vi "ReadCom.vi"(10 "仪器名称":string, 11 "MyIndex":u8) -> (1 "Baudrate":i32, 2 "COM":string, 3 "OK?":bool)   [LabVIEW 2015]
uses:
  <vilib>/Utility/config.llb/Read Key (String).vi
  <vilib>/Utility/config.llb/NI_LVConfig.lvlib
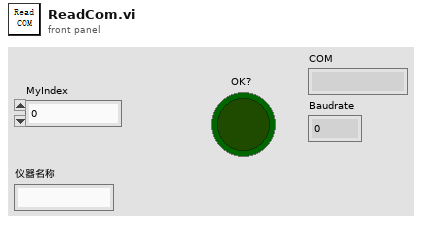
[diagram p1: front panel]
types:
  T1 = typedef "NI_LVConfig.lvlib/Config Data RefNum.ctl" = refnum<k1>
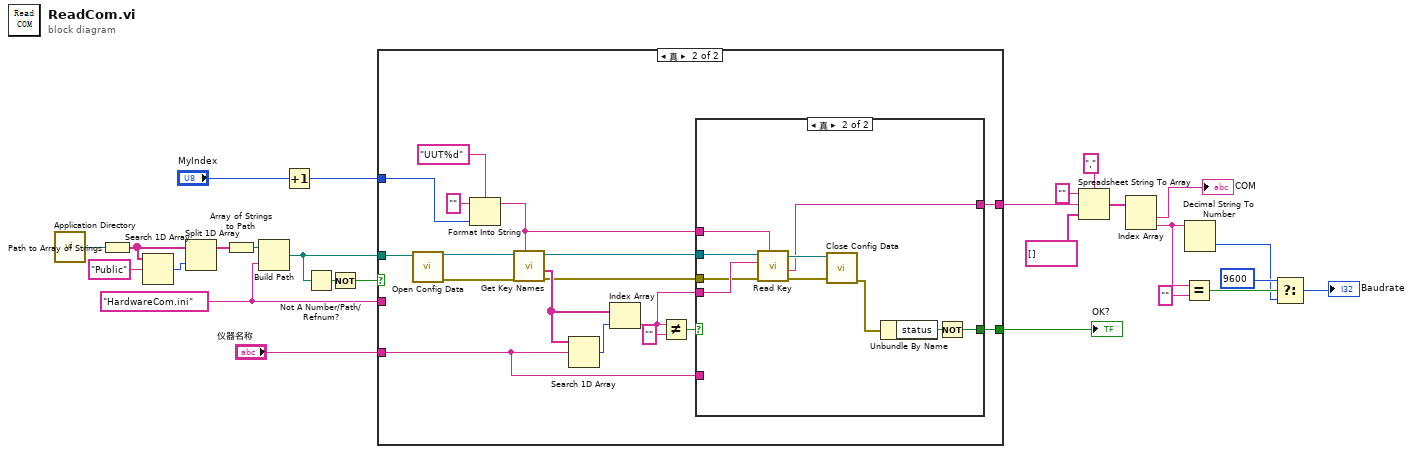
[diagram p0: block diagram]
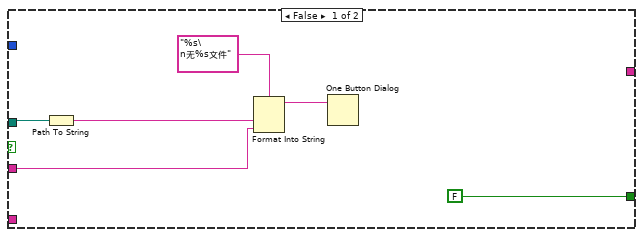
[diagram p2: hidden frame]
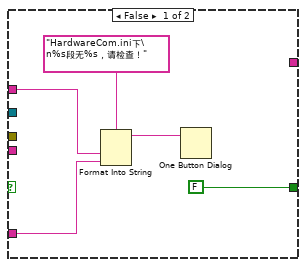
[diagram p3: hidden frame]
diagram:
  w14 = "HardwareCom.ini" ("名称或相对路径")
  n1 = call <vilib>:"Application Directory.vi"() -> ("Application Directory"=w26:path)
  n2 = Path to Array of Strings(0:w26) -> (2:w24:string[])  [unwired: 1 out]
  n3 = Search 1D Array(1D array=w24, element="Public" ("元素")) -> (index of element=w23:i32)  [unwired: 1 in]
  n4 = Split 1D Array(array=w24, index=w23) -> (first subarray=w22:string[])  [unwired: 1 out]
  n5 = Array of Strings to Path(0:w22) -> (2:w21:path)  [unwired: 1 in]
  n6 = Build Path(base path=w21, name or relative path=w14) -> (appended path=w18:path)
  n7 = Increment(x="MyIndex") -> (x+1=w15:u8)
  n8 = Not A Number/Path/Refnum?(number/path/refnum=w18) -> (NaN/Path/Refnum?=w20:bool)
  n9 = Not(x=w20) -> (.not. x?=w19:bool)
  n10 = case shown="真" w19 {
    tunnel: w18 -> [w31 w49]
    tunnel: w15 -> [_ w41]
    tunnel: "仪器名称" -> [_ w39]
    tunnel: w14 -> [w29 _]
    tunnel: [FALSE w37] -> w13
    tunnel: [_ w33] -> w11
    frame False {
      n11 = Path To String(path=w31) -> (string=w30:string)
      n12 = Format Into String(format string="%s\n无%s文件" ("消息"), w30, w29) -> (resulting string=w28:string)  [unwired: 2 in, 1 out]
      n13 = One Button Dialog(message=w28) -> ()  [unwired: 1 in, 1 out]
    }
    frame True {
      n14 = call <vilib>:"Open Config Data.vi"("configuration file path"=w49) -> ("error out"=w47:errorcluster, "refnum"=w48:T1)  [unwired: 8 in, 1 out]
      n15 = Format Into String(format string="UUT%d" ("section"), initial string="" ("初始字符串"), w41) -> (resulting string=w40:string)  [unwired: 1 in, 1 out]
      n16 = call <vilib>:"Get Key Names.vi"("section"=w40, "error in (no error)"=w47, "refnum"=w48) -> ("error out"=w34:errorcluster, "key names"=w44:string[], "refnum out"=w35:T1)  [unwired: 5 in, 1 out]
      n17 = Search 1D Array(1D array=w44, element=w39) -> (index of element=w43:i32)  [unwired: 1 in]
      n18 = Index Array(array=w44, index=w43) -> (element=w36:string)
      n19 = Not Equal?(x=w36, y="") -> (x != y?=w38:bool)
      n20 = case shown="真" w38 {
        tunnel: w40 -> [w53 w64]
        tunnel: w39 -> [w52 _]
        tunnel: [FALSE w56] -> w37
        tunnel: w36 -> [_ w63]
        tunnel: w35 -> [_ w62]
        tunnel: w34 -> [_ w61]
        tunnel: [_ w55] -> w33
        frame False {
          n21 = Format Into String(format string="HardwareCom.ini下\n%s段无%s，请检查！", w53, w52) -> (resulting string=w51:string)  [unwired: 2 in, 1 out]
          n22 = One Button Dialog(message=w51) -> ()  [unwired: 1 in, 1 out]
        }
        frame True {
          n23 = call-poly <vilib>:"Read Key.vi"("section"=w64, "error in (no error)"=w61, "key"=w63, "refnum"=w62) -> ("error out"=w59:errorcluster, "value"=w55:string, "refnum out"=w60:T1)  [unwired: 4 in, 1 out]
          n24 = call <vilib>:"Close Config Data.vi"("error in (no error)"=w59, "refnum"=w60) -> ("error out"=w58:errorcluster)  [unwired: 8 in, 1 out]
          n25 = Unbundle By Name(w58) -> ("status"=w57:bool)
          n26 = Not(x=w57) -> (.not. x?=w56:bool)
        }
      }
    }
  }
  "OK?" <- w13
  n27 = Spreadsheet String To Array(delimiter (Tab)="," ("分隔符(Tab)"), format string="" ("格式字符串"), spreadsheet string=w11, array type (2D Dbl)=string[] []) -> (array=w8:string[])
  n28 = Index Array(array=w8) -> (element #1=→"COM":string, element #2=w6:string)  [unwired: 2 in]
  n29 = Equal?(x=w6, y="") -> (x = y?=w4:bool)
  n30 = Decimal String To Number(string=w6) -> (number=w2:i32)  [unwired: 2 in, 1 out]
  n31 = Select(t=9600, s=w4, f=w2) -> (s? t:f=→"Baudrate":i32)
